vi "Set Up Dialog - Thermistor.vi"() -> ()   [LabVIEW 2012]
panel:
  out "Calibration Instructions":string="1. Connect the sensor to your myDAQ as shown in the diagram above.\n\n2. Prepare 2 water baths, one at 30oC and the other at 40oC. \n\n3. Put the TMN-100 in the 30°C bath first. Once the trace settles record the voltage for SP1.\n\n4. Put the TMN-100 in the 40°C bath. Once the trace settles recrod the voltage for SP2.\n"
  # "iWorx - Thermistor - Set Up"
  # "Temperature (TMN - 100)"
  # "iWorx"
  # "Sensor"
  # "TMN - 100"
  # "myDAQ"
  # "Computer"
  # "Adaptor"
  # "Connection Diagram"
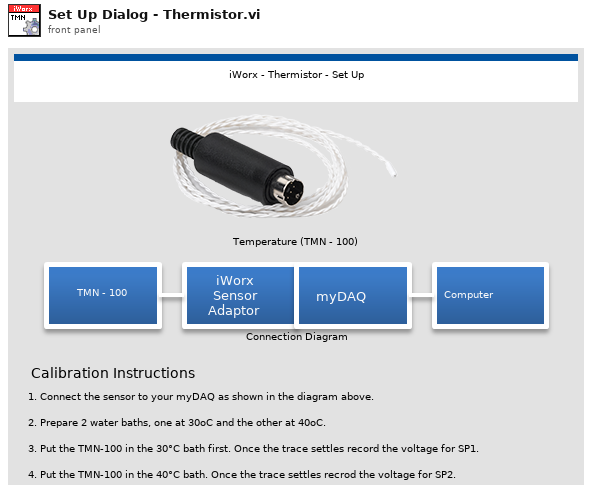
[diagram p1: front panel]
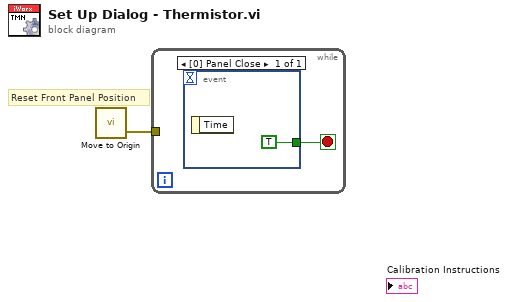
[diagram p0: block diagram]
diagram:
  # "Reset Front Panel Position"
  n1 = call "Move to Origin.vi"() -> ("Error Out"=w1:errorcluster)  [unwired: 3 in]
  n2 = while {
    tunnel: w1 -> [_]
    stop <- w2 stop-if-true
    n3 = event shown="[0] Panel Close" {
      selector: _ -> [_]
      dyn-events: _ -> [_]
      timeout: _ -> [_]
      tunnel: [TRUE] -> w2
      event Panel Close {
        n4 = event-data() -> ()  [unwired: 1 in, 1 out]
      }
    }
  }
